vi "Write Max History.vi"(8 "error in (no error)":errorcluster, 10 "Max History":i32=-1, 11 "Stats_DBL_CIF_U in":refnum<class "Stats_DBL_CIF_U.lvclass">) -> (0 "error out":errorcluster, 3 "Stats_DBL_CIF_U out":refnum<class "Stats_DBL_CIF_U.lvclass">)   [LabVIEW 2021, in "Stats_CIF_U.lvlib" / "Stats_DBL_CIF_U.lvclass"]
doc: "The History sets the maximum number of data points that are used in the rolling average. -1 indicates no limit to the history."
uses:
  Stats_DBL_CIF_U.lvclass
  Stats_DBL_CIF_U.lvclass/Stats_DBL_CIF_U.ctl
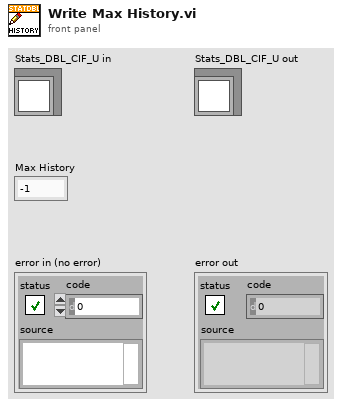
[diagram p1: front panel]
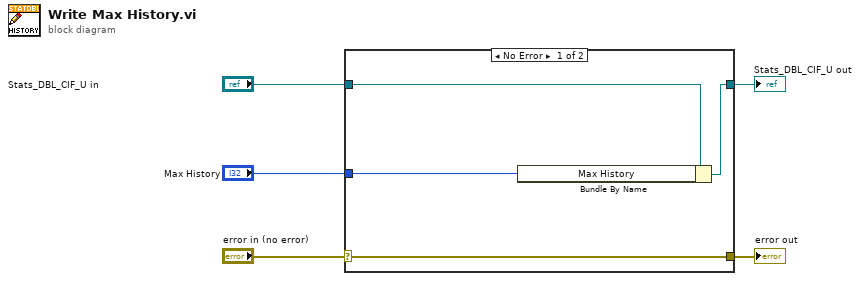
[diagram p0: block diagram]
diagram:
  n1 = case shown="No Error" "error in (no error)" {
    selector: "error in (no error)" -> [w9 w10]
    tunnel: [w9 w10] -> w4
    tunnel: [w7 w11] -> w2
    tunnel: "Stats_DBL_CIF_U in" -> [w8 w11]
    tunnel: "Max History" -> [w6 _]
    frame No Error {
      n2 = Bundle By Name(cluster=w8, "Max History"=w6) -> (w7:refnum<class "Stats_DBL_CIF_U.lvclass">)
    }
    frame Error {
    }
  }
  "error out" <- w4
  "Stats_DBL_CIF_U out" <- w2
